vi "ActionSCPICommand.vi"(8 "error in (no error)":errorcluster, 9 "DigitalOuts":T1, 10 "Analogs":T2, 11 "SCPI":string) -> (0 "error out":errorcluster, 3 "OutputMessage":string)   [LabVIEW 2020]
uses:
  Controls/Analogs.ctl
  Controls/DigitalOuts.ctl
  Controls/DisplayQCommand.ctl
  Controls/DisplayMessage.ctl
  <vilib>/Utility/error.llb/Trim Whitespace One-Sided.vi
  Globals/HandsOnGlobals.vi
panel:
  # "Output"
  # "Input"
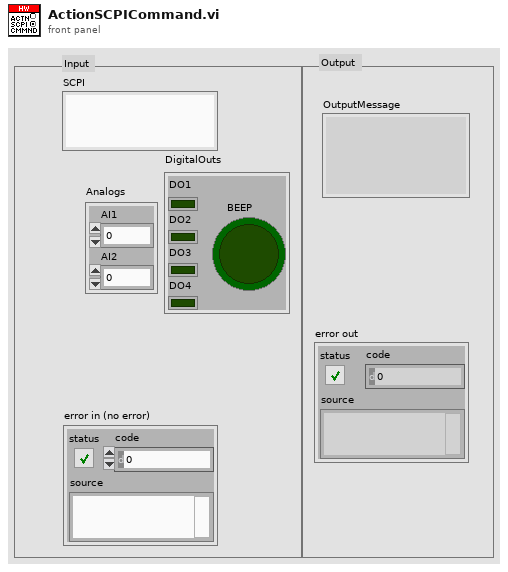
[diagram p1: front panel]
types:
  T1 = typedef "DigitalOuts.ctl" = cluster{"DO1":bool, "DO2":bool, "DO3":bool, "DO4":bool, "BEEP":bool}
  T2 = typedef "Analogs.ctl" = cluster{"AI1":u16, "AI2":u16}
  T3 = typedef "DisplayMessage.ctl" = enum16{"No Message - Ignore", "Display Message", "Set Tab", "Set Status", "Add Error Message", "Clear Error History", "Generate Error", "Set Idling Display", "Set Running Display", "Set DO1", "Set DO2", "Set DO3", "Set DO4", "Set AI1", "Set BEEP", "Update SCPI Return", "Clear SCPI", "Reset Screen", "Set PWM Duty", "Set PWM Freq", "Stop"}
  T4 = typedef "DisplayQCommand.ctl" = enum16{"No Command - Error", "Initialise", "Get Q Reference", "Add Item to Bottom", "Add Item to Top", "Flush Q", "Dequeue", "Peek Next Element", "Close"}
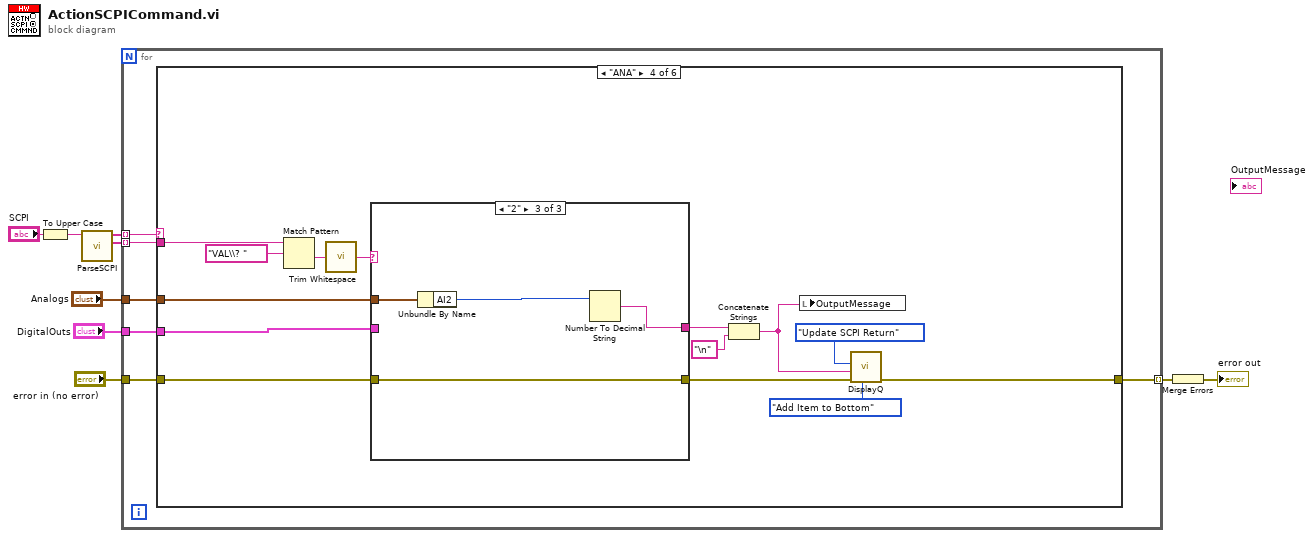
[diagram p0: block diagram]
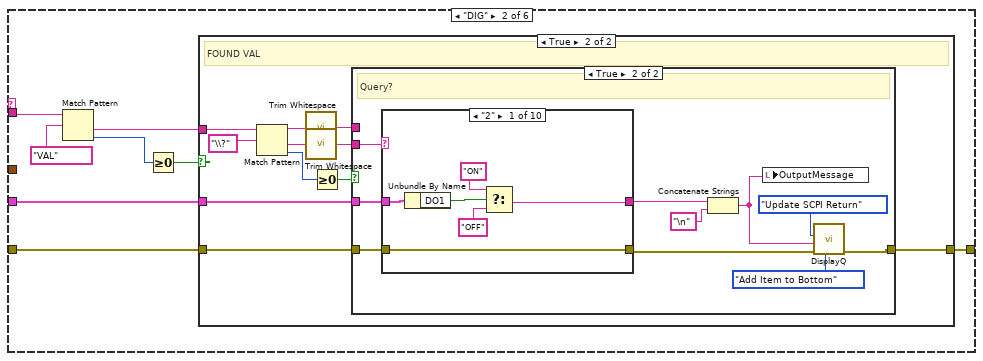
[diagram p3: hidden frame]
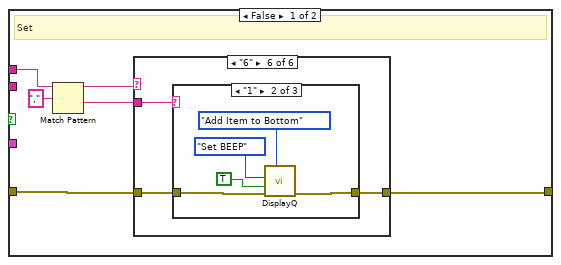
[diagram p5: hidden frame]
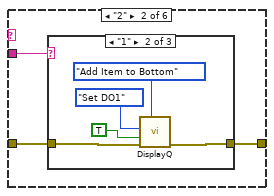
[diagram p7: hidden frame]
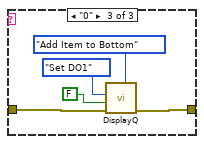
[diagram p9: hidden frame]
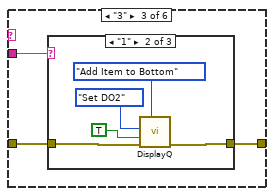
[diagram p10: hidden frame]
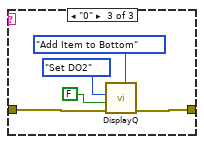
[diagram p12: hidden frame]
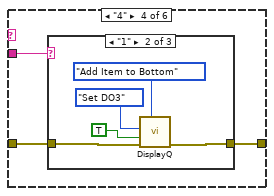
[diagram p13: hidden frame]
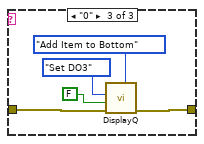
[diagram p15: hidden frame]
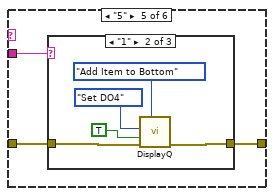
[diagram p16: hidden frame]
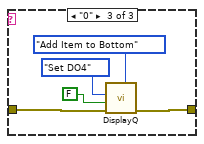
[diagram p18: hidden frame]
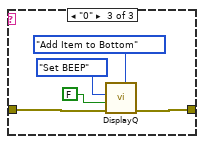
[diagram p20: hidden frame]
diagram:
  n1 = To Upper Case(1:"SCPI") -> (0:w1:string)
  n2 = call "ParseSCPI.vi"("Input String"=w1) -> ("Data Out"=w7:string[], "Commands Out"=w8:string[])  [unwired: 9 in]
  n3 = for {
    tunnel: w8 -> [w15] mode=indexing
    tunnel: w7 -> [w14] mode=indexing
    tunnel: "error in (no error)" -> [w13]
    tunnel: [w12] -> w5 mode=indexing
    tunnel: "Analogs" -> [w11]
    tunnel: "DigitalOuts" -> [w10]
    n4 = case shown="\"ANA\"" w15 {
      tunnel: w14 -> [_ w20 w175 w253 _ _]
      tunnel: w13 -> [w16 w24 w181 w244 w268 w272]
      tunnel: [w16 w23 w180 w249 w270 w274] -> w12
      tunnel: w11 -> [_ _ _ w246 _ _]
      tunnel: w10 -> [_ w22 _ w245 _ _]
      frame "False", Default {
      }
      frame "DIG" {
        n5 = Match Pattern(string=w20, regular expression="VAL") -> (after substring=w19:string, offset past match=w18:i32)  [unwired: 1 in, 2 out]
        n6 = Greater Or Equal To 0?(x=w18) -> (x >= 0?=w17:bool)
        n7 = case shown="True" w17 {
          tunnel: w24 -> [w25 w36]
          tunnel: [w25 w35] -> w23
          tunnel: w22 -> [_ w34]
          tunnel: w19 -> [_ w33]
          frame False {
            # "Unrecognised command"
          }
          frame True {
            # "FOUND VAL"
            n8 = Match Pattern(string=w33, regular expression="\\?") -> (before substring=w27:string, after substring=w31:string, offset past match=w29:i32)  [unwired: 1 in, 1 out]
            n9 = call <vilib>:"Trim Whitespace.vi"("string"=w27) -> ("trimmed string"=w26:string)  [unwired: 1 in]
            n10 = call <vilib>:"Trim Whitespace.vi"("string"=w31) -> ("trimmed string"=w30:string)  [unwired: 1 in]
            n11 = Greater Or Equal To 0?(x=w29) -> (x >= 0?=w28:bool)
            n12 = case shown="True" w28 {
              tunnel: w36 -> [w42 w123]
              tunnel: [w41 w116] -> w35
              tunnel: w34 -> [_ w122]
              tunnel: w30 -> [_ w121]
              tunnel: w26 -> [w37 _]
              frame False {
                # "Set"
                n13 = Match Pattern(string=w37, regular expression=",") -> (before substring=w38:string, after substring=w39:string)  [unwired: 1 in, 2 out]
                n14 = case shown="\"6\"" w38 {
                  tunnel: w42 -> [w43 w46 w60 w74 w88 w102]
                  tunnel: [w43 w45 w59 w73 w87 w101] -> w41
                  tunnel: w39 -> [_ w44 w58 w72 w86 w100]
                  frame "False", Default {
                  }
                  frame "2" {
                    n15 = case shown="\"1\"" w44 {
                      tunnel: w46 -> [w47 w49 w55]
                      tunnel: [w47 w50 w54] -> w45
                      frame "False", Default {
                      }
                      frame "1" {
                        n16 = call "DisplayQ.vi"("command"=DisplayQCommand."Add Item to Bottom", "error in (no error)"=w49, "DataIn"=TRUE, "DisplayMessage"=DisplayMessage."Set DO1") -> ("error out"=w50:errorcluster)  [unwired: 1 in, 3 out]
                      }
                      frame "0" {
                        n17 = call "DisplayQ.vi"("command"=DisplayQCommand."Add Item to Bottom", "error in (no error)"=w55, "DataIn"=FALSE, "DisplayMessage"=DisplayMessage."Set DO1") -> ("error out"=w54:errorcluster)  [unwired: 1 in, 3 out]
                      }
                    }
                  }
                  frame "3" {
                    n18 = case shown="\"1\"" w58 {
                      tunnel: w60 -> [w61 w63 w69]
                      tunnel: [w61 w64 w68] -> w59
                      frame "False", Default {
                      }
                      frame "1" {
                        n19 = call "DisplayQ.vi"("command"=DisplayQCommand."Add Item to Bottom", "error in (no error)"=w63, "DataIn"=TRUE, "DisplayMessage"=DisplayMessage."Set DO2") -> ("error out"=w64:errorcluster)  [unwired: 1 in, 3 out]
                      }
                      frame "0" {
                        n20 = call "DisplayQ.vi"("command"=DisplayQCommand."Add Item to Bottom", "error in (no error)"=w69, "DataIn"=FALSE, "DisplayMessage"=DisplayMessage."Set DO2") -> ("error out"=w68:errorcluster)  [unwired: 1 in, 3 out]
                      }
                    }
                  }
                  frame "4" {
                    n21 = case shown="\"1\"" w72 {
                      tunnel: w74 -> [w75 w77 w83]
                      tunnel: [w75 w78 w82] -> w73
                      frame "False", Default {
                      }
                      frame "1" {
                        n22 = call "DisplayQ.vi"("command"=DisplayQCommand."Add Item to Bottom", "error in (no error)"=w77, "DataIn"=TRUE, "DisplayMessage"=DisplayMessage."Set DO3") -> ("error out"=w78:errorcluster)  [unwired: 1 in, 3 out]
                      }
                      frame "0" {
                        n23 = call "DisplayQ.vi"("command"=DisplayQCommand."Add Item to Bottom", "error in (no error)"=w83, "DataIn"=FALSE, "DisplayMessage"=DisplayMessage."Set DO3") -> ("error out"=w82:errorcluster)  [unwired: 1 in, 3 out]
                      }
                    }
                  }
                  frame "5" {
                    n24 = case shown="\"1\"" w86 {
                      tunnel: w88 -> [w89 w91 w97]
                      tunnel: [w89 w92 w96] -> w87
                      frame "False", Default {
                      }
                      frame "1" {
                        n25 = call "DisplayQ.vi"("command"=DisplayQCommand."Add Item to Bottom", "error in (no error)"=w91, "DataIn"=TRUE, "DisplayMessage"=DisplayMessage."Set DO4") -> ("error out"=w92:errorcluster)  [unwired: 1 in, 3 out]
                      }
                      frame "0" {
                        n26 = call "DisplayQ.vi"("command"=DisplayQCommand."Add Item to Bottom", "error in (no error)"=w97, "DataIn"=FALSE, "DisplayMessage"=DisplayMessage."Set DO4") -> ("error out"=w96:errorcluster)  [unwired: 1 in, 3 out]
                      }
                    }
                  }
                  frame "6" {
                    n27 = case shown="\"1\"" w100 {
                      tunnel: w102 -> [w103 w105 w111]
                      tunnel: [w103 w106 w110] -> w101
                      frame "False", Default {
                      }
                      frame "1" {
                        n28 = call "DisplayQ.vi"("command"=DisplayQCommand."Add Item to Bottom", "error in (no error)"=w105, "DataIn"=TRUE, "DisplayMessage"=DisplayMessage."Set BEEP") -> ("error out"=w106:errorcluster)  [unwired: 1 in, 3 out]
                      }
                      frame "0" {
                        n29 = call "DisplayQ.vi"("command"=DisplayQCommand."Add Item to Bottom", "error in (no error)"=w111, "DataIn"=FALSE, "DisplayMessage"=DisplayMessage."Set BEEP") -> ("error out"=w110:errorcluster)  [unwired: 1 in, 3 out]
                      }
                    }
                  }
                }
              }
              frame True {
                # "Query?"
                n30 = case shown="\"2\"" w121 {
                  tunnel: [w126 w133 w139 w145 w150 w156 w161 w166 w171 w174] -> w115
                  tunnel: [w124 w130 w136 w142 w148 w155 w160 w165 w170 _] -> w114
                  tunnel: w123 -> [w126 w133 w139 w145 w150 w156 w161 w166 w171 w174]
                  tunnel: w122 -> [w125 w131 w137 w143 w149 _ _ _ _ _]
                  frame "2" {
                    n31 = Unbundle By Name(w125) -> ("DO1"=w128:bool)
                    n32 = Select(t="ON", s=w128, f="OFF") -> (s? t:f=w124:string)
                  }
                  frame "3" {
                    n33 = Unbundle By Name(w131) -> ("DO2"=w134:bool)
                    n34 = Select(t="ON", s=w134, f="OFF") -> (s? t:f=w130:string)
                  }
                  frame "4" {
                    n35 = Unbundle By Name(w137) -> ("DO3"=w140:bool)
                    n36 = Select(t="ON", s=w140, f="OFF") -> (s? t:f=w136:string)
                  }
                  frame "5" {
                    n37 = Unbundle By Name(w143) -> ("DO4"=w146:bool)
                    n38 = Select(t="ON", s=w146, f="OFF") -> (s? t:f=w142:string)
                  }
                  frame "6" {
                    n39 = Unbundle By Name(w149) -> ("BEEP"=w152:bool)
                    n40 = Select(t="ON", s=w152, f="OFF") -> (s? t:f=w148:string)
                  }
                  frame "7" {
                    n41 = global read "HandsOnGlobals.vi" "DI 1 Pressed"() -> (w154:bool)
                    n42 = Select(t="OFF", s=w154, f="ON") -> (s? t:f=w155:string)
                  }
                  frame "8" {
                    n43 = global read "HandsOnGlobals.vi" "DI 2 Pressed"() -> (w159:bool)
                    n44 = Select(t="OFF", s=w159, f="ON") -> (s? t:f=w160:string)
                  }
                  frame "9" {
                    n45 = global read "HandsOnGlobals.vi" "DI 3 Pressed"() -> (w164:bool)
                    n46 = Select(t="OFF", s=w164, f="ON") -> (s? t:f=w165:string)
                  }
                  frame "10" {
                    n47 = global read "HandsOnGlobals.vi" "DI 4 Pressed"() -> (w169:bool)
                    n48 = Select(t="OFF", s=w169, f="ON") -> (s? t:f=w170:string)
                  }
                  frame "False", Default {
                  }
                }
                n49 = Concatenate Strings(w114, "\n" ("string")) -> (w120:string)
                n50 = local write "OutputMessage"(w120) -> ()
                n51 = call "DisplayQ.vi"("command"=DisplayQCommand."Add Item to Bottom", "error in (no error)"=w115, "DataIn"=w120, "DisplayMessage"=DisplayMessage."Update SCPI Return") -> ("error out"=w116:errorcluster)  [unwired: 1 in, 3 out]
              }
            }
          }
        }
      }
      frame "PWM" {
        n52 = Match Pattern(string=w175, regular expression="DUTY") -> (after substring=w178:string, offset past match=w177:i32)  [unwired: 1 in, 2 out]
        n53 = Greater Or Equal To 0?(x=w177) -> (x >= 0?=w176:bool)
        n54 = case shown="True" w176 {
          tunnel: w181 -> [w188 w224]
          tunnel: [w187 w223] -> w180
          tunnel: w178 -> [_ w222]
          tunnel: w175 -> [w185 _]
          frame False {
            # "Unrecognised command"
            n55 = Match Pattern(string=w185, regular expression="FREQ") -> (after substring=w182:string, offset past match=w184:i32)  [unwired: 1 in, 2 out]
            n56 = Greater Or Equal To 0?(x=w184) -> (x >= 0?=w183:bool)
            n57 = case shown="True" w183 {
              tunnel: w188 -> [w189 w192]
              tunnel: [w189 w191] -> w187
              tunnel: w182 -> [_ w190]
              frame False {
                # "Unrecognised command"
              }
              frame True {
                # "FOUND FREQ"
                n58 = Match Pattern(string=w190, regular expression="\\?") -> (before substring=w194:string, after substring=w198:string, offset past match=w196:i32)  [unwired: 1 in, 1 out]
                n59 = call <vilib>:"Trim Whitespace.vi"("string"=w194) -> ("trimmed string"=w193:string)  [unwired: 1 in]
                n60 = call <vilib>:"Trim Whitespace.vi"("string"=w198) -> ("trimmed string"=w197:string)  [unwired: 1 in]
                n61 = Greater Or Equal To 0?(x=w196) -> (x >= 0?=w195:bool)
                n62 = case shown="True" w195 {
                  tunnel: w192 -> [w206 w210]
                  tunnel: [w205 w209] -> w191
                  tunnel: w197 -> [_ _]
                  tunnel: w193 -> [w202 _]
                  frame False {
                    # "Set"
                    n63 = Scan From String(format string="%f,%f", input string=w202) -> (output 2=w200:dbl)  [unwired: 5 in, 3 out]
                    n64 = call "DisplayQ.vi"("command"=DisplayQCommand."Add Item to Bottom", "error in (no error)"=w206, "DataIn"=w200, "DisplayMessage"=DisplayMessage."Set PWM Freq") -> ("error out"=w205:errorcluster)  [unwired: 1 in, 3 out]
                  }
                  frame True {
                    # "Query?"
                    n65 = global read "HandsOnGlobals.vi" "PWMFreq"() -> (w208:dbl)
                    n66 = Number To Fractional String(number=w208) -> (F-format string=w211:string)  [unwired: 3 in]
                    n67 = Concatenate Strings(w211, "\n" ("string")) -> (w207:string)
                    n68 = local write "OutputMessage"(w207) -> ()
                    n69 = call "DisplayQ.vi"("command"=DisplayQCommand."Add Item to Bottom", "error in (no error)"=w210, "DataIn"=w207, "DisplayMessage"=DisplayMessage."Update SCPI Return") -> ("error out"=w209:errorcluster)  [unwired: 1 in, 3 out]
                  }
                }
              }
            }
          }
          frame True {
            # "FOUND DUTY"
            n70 = Match Pattern(string=w222, regular expression="\\?") -> (before substring=w216:string, after substring=w220:string, offset past match=w218:i32)  [unwired: 1 in, 1 out]
            n71 = call <vilib>:"Trim Whitespace.vi"("string"=w216) -> ("trimmed string"=w215:string)  [unwired: 1 in]
            n72 = call <vilib>:"Trim Whitespace.vi"("string"=w220) -> ("trimmed string"=w219:string)  [unwired: 1 in]
            n73 = Greater Or Equal To 0?(x=w218) -> (x >= 0?=w217:bool)
            n74 = case shown="True" w217 {
              tunnel: w224 -> [w231 w236]
              tunnel: [w230 w237] -> w223
              tunnel: w219 -> [_ _]
              tunnel: w215 -> [w227 _]
              frame False {
                # "Set"
                n75 = Scan From String(format string="%f,%f", input string=w227) -> (output 2=w225:dbl)  [unwired: 5 in, 3 out]
                n76 = call "DisplayQ.vi"("command"=DisplayQCommand."Add Item to Bottom", "error in (no error)"=w231, "DataIn"=w225, "DisplayMessage"=DisplayMessage."Set PWM Duty") -> ("error out"=w230:errorcluster)  [unwired: 1 in, 3 out]
              }
              frame True {
                # "Query?"
                n77 = global read "HandsOnGlobals.vi" "PWMDuty"() -> (w235:dbl)
                n78 = Number To Fractional String(number=w235) -> (F-format string=w233:string)  [unwired: 3 in]
                n79 = Concatenate Strings(w233, "\n" ("string")) -> (w232:string)
                n80 = local write "OutputMessage"(w232) -> ()
                n81 = call "DisplayQ.vi"("command"=DisplayQCommand."Add Item to Bottom", "error in (no error)"=w236, "DataIn"=w232, "DisplayMessage"=DisplayMessage."Update SCPI Return") -> ("error out"=w237:errorcluster)  [unwired: 1 in, 3 out]
              }
            }
          }
        }
      }
      frame "ANA" {
        n82 = Match Pattern(string=w253, regular expression="VAL\\? ") -> (after substring=w243:string)  [unwired: 1 in, 3 out]
        n83 = call <vilib>:"Trim Whitespace.vi"("string"=w243) -> ("trimmed string"=w251:string)  [unwired: 1 in]
        n84 = case shown="\"2\"" w251 {
          tunnel: [w254 w258 w262] -> w247
          tunnel: [_ w256 w259] -> w241
          tunnel: w246 -> [_ w257 w261]
          tunnel: w245 -> [_ _ _]
          tunnel: w244 -> [w254 w258 w262]
          frame "False", Default {
          }
          frame "1" {
            n85 = Unbundle By Name(w257) -> ("AI1"=w255:u16)
            n86 = Number To Decimal String(number=w255) -> (decimal integer string=w256:string)  [unwired: 1 in]
          }
          frame "2" {
            n87 = Unbundle By Name(w261) -> ("AI2"=w260:u16)
            n88 = Number To Decimal String(number=w260) -> (decimal integer string=w259:string)  [unwired: 1 in]
          }
        }
        n89 = Concatenate Strings(w241, "\n" ("string")) -> (w240:string)
        n90 = local write "OutputMessage"(w240) -> ()
        n91 = call "DisplayQ.vi"("command"=DisplayQCommand."Add Item to Bottom", "error in (no error)"=w247, "DataIn"=w240, "DisplayMessage"=DisplayMessage."Update SCPI Return") -> ("error out"=w249:errorcluster)  [unwired: 1 in, 3 out]
      }
      frame "*IDN?" {
        n92 = call "Version.vi"() -> ("Version"=w267:string)  [unwired: 5 in]
        n93 = Format Into String(format string="CTI,RP2040-Visa,Emulator,%s20230827T193959Z" ("data in"), w267) -> (resulting string=w264:string)  [unwired: 2 in, 1 out]
        n94 = Concatenate Strings(w264, "\n" ("string")) -> (w263:string)
        n95 = local write "OutputMessage"(w263) -> ()
        n96 = call "DisplayQ.vi"("command"=DisplayQCommand."Add Item to Bottom", "error in (no error)"=w268, "DataIn"=w263, "DisplayMessage"=DisplayMessage."Update SCPI Return") -> ("error out"=w270:errorcluster)  [unwired: 1 in, 3 out]
      }
      frame "*RST" {
        n97 = call "DisplayQ.vi"("command"=DisplayQCommand."Add Item to Bottom", "error in (no error)"=w272, "DisplayMessage"=DisplayMessage."Reset Screen") -> ("error out"=w274:errorcluster)  [unwired: 2 in, 3 out]
      }
    }
  }
  n98 = Merge Errors(w5) -> (→"error out":errorcluster)
